vi "SimulateCodeModule.vi"(7 "Simulate Failure":bool, 9 "Message":string, 10 "Test Duration (S)":dbl, 11 "Sequence Context In":refnum<k7>) -> (0 "error out":errorcluster, 3 "Result Out":bool)   [LabVIEW 2011]
panel:
  out "Slide":u8(slide) scale=0.0..100.0
  out "DisplaySocket":i32 caption="Test Socket"
  out "DisplayString":string
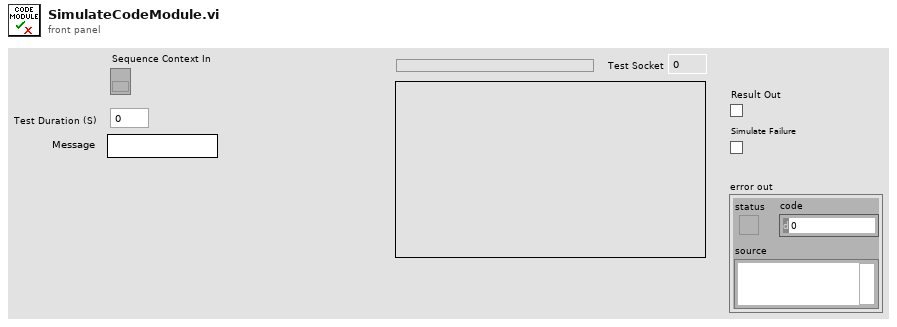
[diagram p1: front panel]
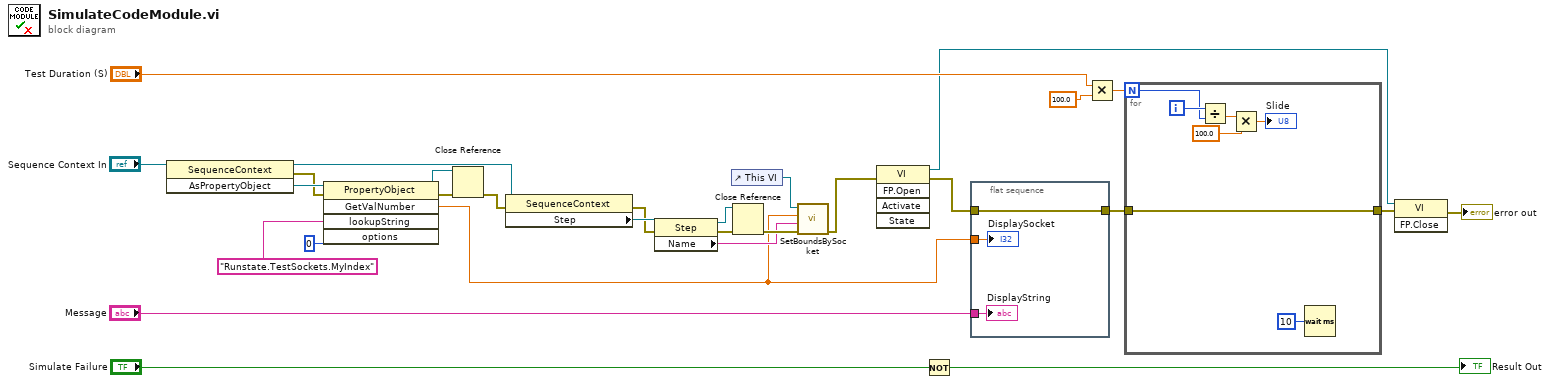
[diagram p0: block diagram]
diagram:
  n1 = invoke class="SequenceContext" method="AsPropertyObject"(reference="Sequence Context In") -> (reference out=w10:refnum<k7>, error out=w14:errorcluster, "AsPropertyObject"=w15:refnum<k7>)  [unwired: 2 in]
  n2 = invoke class="PropertyObject" method="GetValNumber"(reference=w15, error in=w14, "lookupString"="Runstate.TestSockets.MyIndex" ("Lookup String"), "options"=0) -> (reference out=w12:refnum<k7>, error out=w13:errorcluster, "GetValNumber"=w3:dbl)  [unwired: 1 in, 2 out]
  n3 = Close Reference(reference=w12, error in (no error)=w13) -> (error out=w11:errorcluster)
  n4 = property class="SequenceContext"(reference=w10, error in=w11) -> (error out=w19:errorcluster, "Step"=w20:refnum<k7>)  [unwired: 1 out]
  n5 = property class="Step"(reference=w20, error in=w19) -> (reference out=w17:refnum<k7>, error out=w18:errorcluster, "Name"=w4:string)
  n6 = control-ref of="This VI"() -> (w2:refnum<vi>)
  n7 = Close Reference(reference=w17, error in (no error)=w18) -> (error out=w16:errorcluster)
  n8 = call "SetBoundsBySocket.vi"("Error In"=w16, "Test Name"=w4, "Test Socket"=w3, "vi reference"=w2) -> ("Error Out"=w25:errorcluster)  [unwired: 7 in]
  n9 = invoke class="VI" method="FP.Open"(error in=w25) -> (reference out=w21:refnum<vi>, error out=w23:errorcluster)  [unwired: 4 in, 3 out]
  n10 = Not(x="Simulate Failure") -> (.not. x?=→"Result Out":bool)
  n11 = flat-sequence {
    tunnel: "Message" -> [w32]
    tunnel: [w31] -> w24
    tunnel: w23 -> [w31]
    tunnel: w3 -> [w30]
    frame #0 {
      "DisplayString" <- w32
      "DisplaySocket" <- w30
    }
  }
  n12 = Multiply(x="Test Duration (S)", y=100.0) -> (x*y=w27:dbl)
  n13 = for {
    N: w27 -> [w33]
    tunnel: w24 -> [w34]
    tunnel: [w34] -> w22
    i -> [w39]
    n14 = Divide(x=w39, y=w33) -> (x/y=w37:dbl)
    n15 = Multiply(x=w37, y=100.0) -> (x*y=→"Slide":dbl)
    n16 = Wait (ms)(milliseconds to wait=u32 10) -> ()  [unwired: 1 out]
  }
  n17 = invoke class="VI" method="FP.Close"(reference=w21, error in=w22) -> (error out=→"error out":errorcluster)  [unwired: 1 in, 2 out]
